vi "Queue Mailbox New.vi"(6 "Creator":refnum<data-value>, 8 "Creator Alias":string, 9 "Self":refnum<data-value>, 10 "Self Alias":string) -> (0 "error out":errorcluster, 2 "Queue Mailbox":refnum<data-value>)   [LabVIEW 2021, in "jettl.lvlib" / "Mailbox.lvlib"]
uses:
  Mailbox/Mailbox.lvlib
  Queue Mailbox/Queue Mailbox.lvclass
  Msg Strategy/Msg Strategy.lvclass
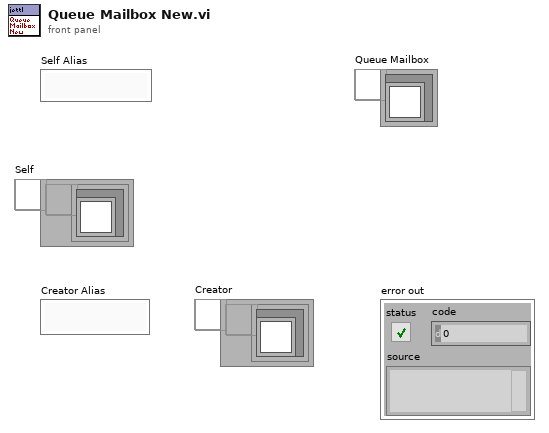
[diagram p1: front panel]
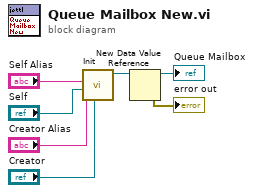
[diagram p0: block diagram]
diagram:
  n1 = call "Init.vi"("Creator"="Creator", "Creator Alias"="Creator Alias", "Self"="Self", "Self Alias"="Self Alias") -> ("Queue Mailbox out"=w1:refnum<class "Queue Mailbox.lvclass">)  [unwired: 7 in]
  n2 = New Data Value Reference(data value=w1) -> (data value reference=→"Queue Mailbox":refnum<data-value>, error out=→"error out":errorcluster)  [unwired: 1 in]
